vi "Check for valid T change.vi"(6 "Max delta":dbl=150.0, 7 "LAB deg C":T1, 8 "T4":dbl, 9 "T3":dbl, 10 "T2":dbl, 11 "T1":dbl) -> (2 "Fault":bool)   [LabVIEW 2017]
panel:
  out "abs(x) 4":dbl
  out "abs(x) 3":dbl
  out "abs(x) 2":dbl
  out "abs(x)1":dbl
  in  "stop":bool
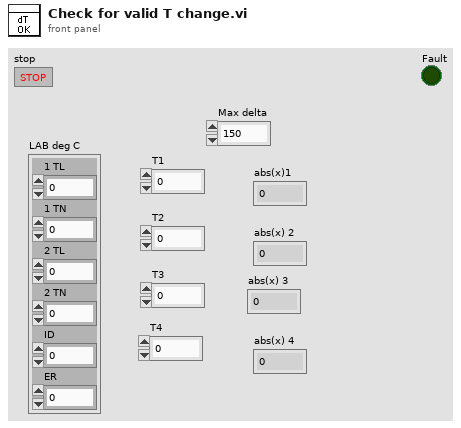
[diagram p1: front panel]
types:
  T1 = cluster{"1 TL":dbl, "1 TN":dbl, "2 TL":dbl, "2 TN":dbl, "ID":dbl, "ER":dbl}
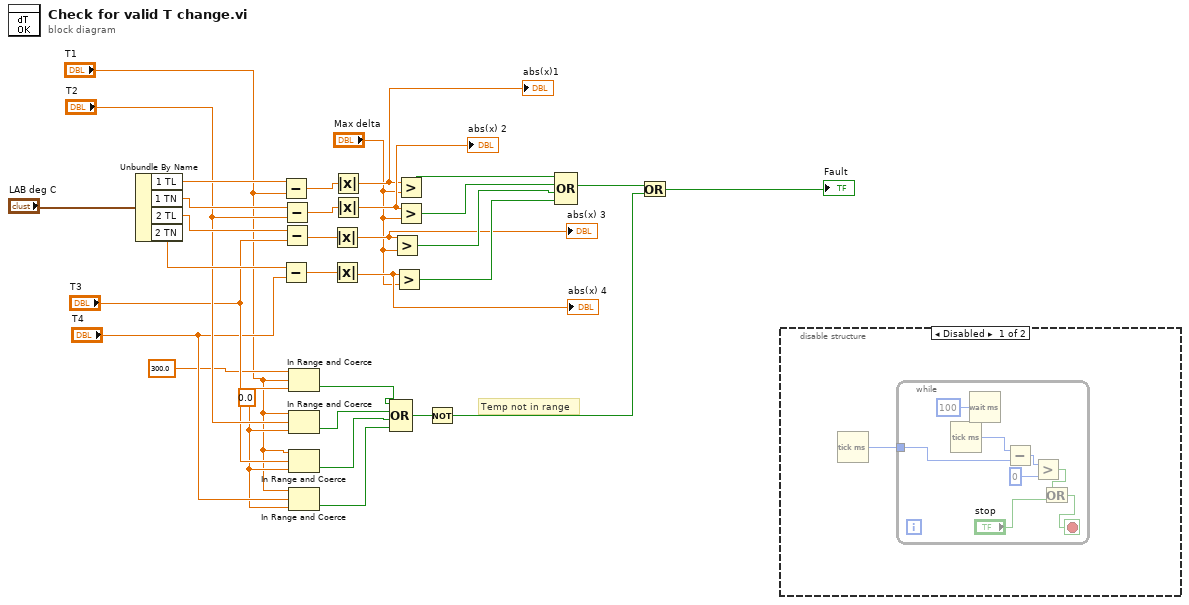
[diagram p0: block diagram]
diagram:
  w12 = 0.0 ("lower limit")
  # "Temp not in range"
  n1 = Unbundle By Name("LAB deg C") -> ("1 TL"=w29:dbl, "1 TN"=w30:dbl, "2 TL"=w31:dbl, "2 TN"=w32:dbl)
  n2 = Subtract(x=w29, y="T1") -> (x-y=w27:dbl)
  n3 = Subtract(x=w32, y="T4") -> (x-y=w24:dbl)
  n4 = Subtract(x=w30, y="T2") -> (x-y=w26:dbl)
  n5 = Subtract(x=w31, y="T3") -> (x-y=w25:dbl)
  n6 = In Range and Coerce(upper limit=300.0, x="T1", lower limit=w12) -> (In Range?=w10:bool)  [unwired: 1 out]
  n7 = In Range and Coerce(upper limit="T1", x="T2", lower limit=w12) -> (In Range?=w9:bool)  [unwired: 1 out]
  n8 = In Range and Coerce(upper limit="T1", x="T3", lower limit=w12) -> (In Range?=w8:bool)  [unwired: 1 out]
  n9 = In Range and Coerce(upper limit="T1", x="T4", lower limit=w12) -> (In Range?=w7:bool)  [unwired: 1 out]
  n10 = Absolute Value(x=w25) -> (abs(x)=w18:dbl)
  "abs(x) 3" <- w18
  n11 = Absolute Value(x=w24) -> (abs(x)=w19:dbl)
  "abs(x) 4" <- w19
  n12 = Absolute Value(x=w27) -> (abs(x)=w16:dbl)
  "abs(x)1" <- w16
  n13 = Absolute Value(x=w26) -> (abs(x)=w17:dbl)
  "abs(x) 2" <- w17
  n14 = Compound Arithmetic op=OR(w10, w9, w8, w7) -> (w5:bool)
  n15 = Greater?(x=w18, y="Max delta") -> (0:w21:bool)
  n16 = Greater?(x=w19, y="Max delta") -> (0:w20:bool)
  n17 = Greater?(x=w16, y="Max delta") -> (0:w23:bool)
  n18 = Greater?(x=w17, y="Max delta") -> (0:w22:bool)
  n19 = Not(x=w5) -> (.not. x?=w4:bool)
  n20 = Compound Arithmetic op=OR(w23, w22, w21, w20) -> (w6:bool)
  n21 = Or(x=w6, y=w4) -> (x .or. y?=→"Fault":bool)
  n22 = disable-structure shown="Disabled" {
    frame Disabled {
      n23 = Tick Count (ms)() -> (millisecond timer value=w33:u32)
      n24 = while {
        tunnel: w33 -> [w39]
        stop <- w34 stop-if-true
        n25 = Tick Count (ms)() -> (millisecond timer value=w40:u32)
        n26 = Wait (ms)(milliseconds to wait=u32 100) -> ()  [unwired: 1 out]
        n27 = Subtract(x=w40, y=w39) -> (x-y=w38:u32)
        n28 = Greater?(x=w38, y=u32 0) -> (0:w36:bool)
        n29 = Or(x=w36, y="stop") -> (x .or. y?=w34:bool)
      }
    }
    frame Enabled {
    }
  }
